vi "Parse.vi"(8 "error in (no error)":errorcluster, 10 "Arguments (From Args)":string[](array[string]), 11 "LV Argument Parser in (Global)":refnum<class "LV Argument Parser.lvclass">) -> (0 "error out":errorcluster, 2 "Output":string, 3 "LV Argument Parser out":refnum<class "LV Argument Parser.lvclass">)   [LabVIEW 2020, in "LV ArgParse.lvlib" / "LV Argument Parser.lvclass"]
uses:
  LV Argument Parser.lvclass
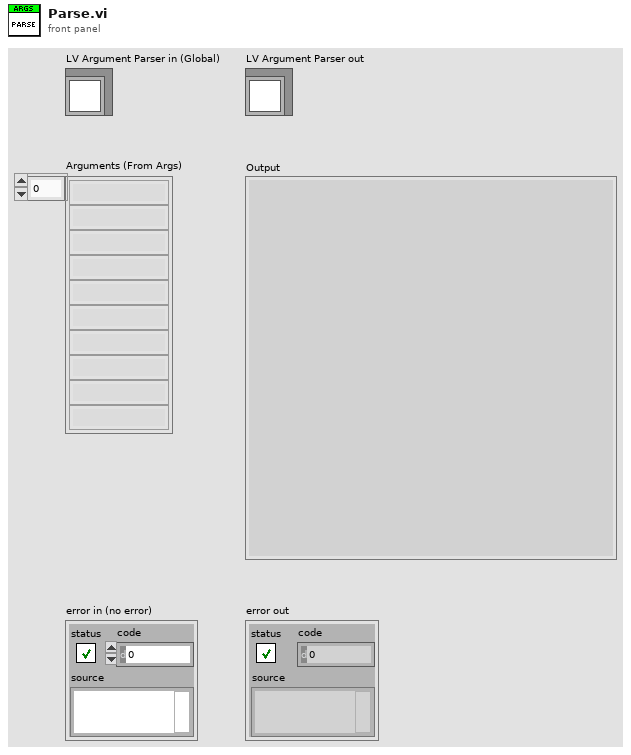
[diagram p1: front panel]
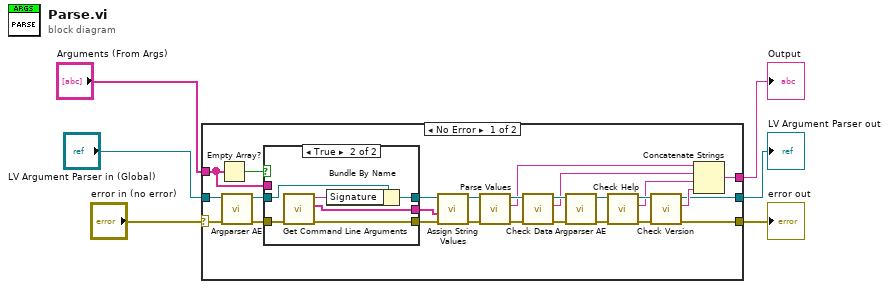
[diagram p0: block diagram]
diagram:
  n1 = case shown="No Error" "error in (no error)" {
    selector: "error in (no error)" -> [w24 w43]
    tunnel: [w15 w43] -> w5
    tunnel: "Arguments (From Args)" -> [w25 _]
    tunnel: [w9 _] -> w3
    tunnel: "LV Argument Parser in (Global)" -> [w8 w42]
    tunnel: [w7 w42] -> w1
    frame No Error {
      n2 = Empty Array?(array=w25) -> (empty?=w27:bool)
      n3 = call "Argparser AE.vi"("error in (no error)"=w24, "LV Argument Parser in"=w8) -> ("error out"=w17:errorcluster, "LV Argument Parser out"=w20:refnum<class "LV Argument Parser.lvclass">)  [unwired: 8 in]
      n4 = case shown="True" w27 {
        tunnel: [w35 w36] -> w26
        tunnel: w25 -> [w35 _]
        tunnel: w17 -> [w34 w41]
        tunnel: [w34 w38] -> w23
        tunnel: w20 -> [w33 w40]
        tunnel: [w33 w39] -> w19
        frame False {
        }
        frame True {
          n5 = call <vilib>:"Get Command Line Arguments.vi"("error in (no error)"=w41) -> ("error out"=w38:errorcluster, "arguments"=w36:string[], "application name"=w37:string)  [unwired: 8 in]
          n6 = Bundle By Name(cluster=w40, "Signature"=w37) -> (w39:refnum<class "LV Argument Parser.lvclass">)
        }
      }
      n7 = call "Assign String Values.vi"("error in (no error)"=w23, "Arguments"=w26, "LV Argument Parser in"=w19) -> ("error IO"=w30:errorcluster, "LV Argument Parser out"=w32:refnum<class "LV Argument Parser.lvclass">)  [unwired: 7 in]
      n8 = call "Parse Values.vi"("error in"=w30, "LV Argument Parser in"=w32) -> ("error out"=w29:errorcluster, "Output"=w13:string, "LV Argument Parser out"=w31:refnum<class "LV Argument Parser.lvclass">)  [unwired: 7 in]
      n9 = call "Check Data.vi"("error IO"=w29, "LV Argument Parser in"=w31) -> ("error out"=w28:errorcluster, "Output"=w12:string, "LV Argument Parser out"=w21:refnum<class "LV Argument Parser.lvclass">)  [unwired: 7 in]
      n10 = call "Argparser AE.vi"("error in (no error)"=w28, "LV Argument Parser in"=w21) -> ("error out"=w22:errorcluster, "LV Argument Parser out"=w18:refnum<class "LV Argument Parser.lvclass">)  [unwired: 8 in]
      n11 = call "Check Help.vi"("error in (no error)"=w22, "LV Argument Parser in"=w18) -> ("error out"=w16:errorcluster, "Output"=w11:string, "LV Argument Parser out"=w14:refnum<class "LV Argument Parser.lvclass">)  [unwired: 7 in]
      n12 = call "Check Version.vi"("error in (no error)"=w16, "LV Argument Parser in"=w14) -> ("error out"=w15:errorcluster, "Output"=w10:string, "LV Argument Parser out"=w7:refnum<class "LV Argument Parser.lvclass">)  [unwired: 7 in]
      n13 = Concatenate Strings(w13, w12, w11, w10) -> (w9:string)
    }
    frame Error {
    }
  }
  "error out" <- w5
  "Output" <- w3
  "LV Argument Parser out" <- w1
